vi "Log Error.vi"(7 "Source":string, 8 "error in (no error)":errorcluster, 10 "Message":string, 11 "Logging In":refnum<class "Logging.lvclass">) -> (0 "error out":errorcluster, 3 "Logging Out":refnum<class "Logging.lvclass">)   [LabVIEW 2021, in "Logging.lvclass"]
doc: "Enter an error-level message into the system log.\nAn error occurs due to a more serious problem, the software has not been able to perform some function.\nLogging is not meant as a substitute for error handling."
uses:
  Logging.lvclass
  Protected/Level.ctl
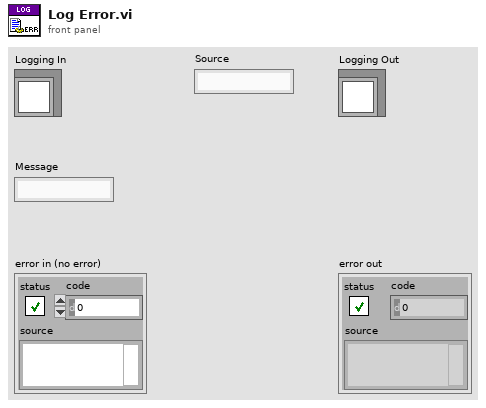
[diagram p1: front panel]
types:
  T1 = typedef "Logging.lvclass/Level.ctl" = enum16{"DEBUG", "INFO", "WARNING", "ERROR", "CRITICAL"}
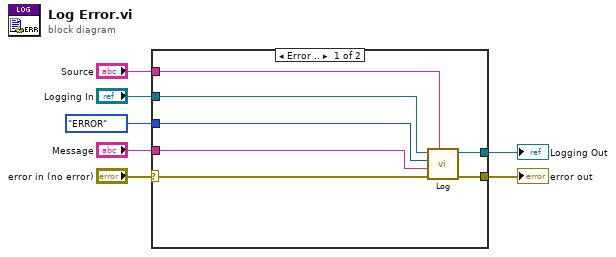
[diagram p0: block diagram]
diagram:
  n1 = case shown="Error .." "error in (no error)" {
    selector: "error in (no error)" -> [w10 w15]
    tunnel: [w14 w15] -> w7
    tunnel: "Logging In" -> [w13 w16]
    tunnel: [w12 w16] -> w5
    tunnel: Level."ERROR" ("Level") -> [w11 _]
    tunnel: "Message" -> [w8 _]
    tunnel: "Source" -> [w9 _]
    frame Error {
      n2 = call-dynamic "Log.vi"("Source"=w9, "error in (no error)"=w10, "Message"=w8, "Level"=w11, "Logging In"=w13) -> ("error out"=w14:errorcluster, "Logging Out"=w12:refnum<class "Logging.lvclass">)  [unwired: 5 in]
    }
    frame No Error {
    }
  }
  "error out" <- w7
  "Logging Out" <- w5
